vi "IoT_GetFileName.vi"() -> (3 "FileName":string)   [LabVIEW 2016]
panel:
  out "call chain":string[](array[string])
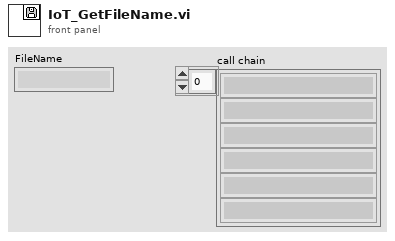
[diagram p1: front panel]
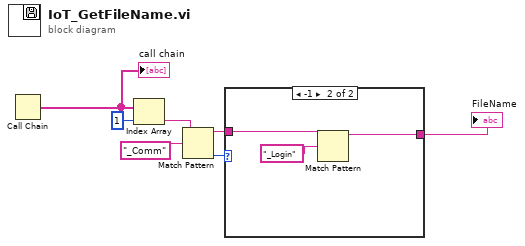
[diagram p0: block diagram]
diagram:
  n1 = Call Chain() -> (call chain=w6:string[])
  "call chain" <- w6
  n2 = Index Array(array=w6, index=1) -> (element=w7:string)
  n3 = Match Pattern(string=w7, regular expression="_Comm") -> (before substring=w2:string, offset past match=w3:i32)  [unwired: 1 in, 2 out]
  n4 = case shown="-1" w3 {
    tunnel: w2 -> [w8 w10]
    tunnel: [w8 w9] -> w1
    frame 0, Default {
    }
    frame -1 {
      n5 = Match Pattern(string=w10, regular expression="_Login") -> (before substring=w9:string)  [unwired: 1 in, 3 out]
    }
  }
  "FileName" <- w1
